vi "Pre Launch Init.vi"(11 "ATM-Controller in":refnum<class "ATM-Controller.lvclass">) -> (0 "error out":errorcluster, 3 "ATM-Controller out":refnum<class "ATM-Controller.lvclass">)   [LabVIEW 2025, in "ATM-Controller.lvlib" / "ATM-Controller.lvclass"]
doc: "<p>(<strong>Filename</strong>: <span class=\"dnl\">Actor Framework.lvlib:Actor.lvclass:Pre Launch Init.vi</span>)</p>\n<p>Defines behavior that occurs after the <a href=\"nihelplauncher://docs/csh?context=lvcore_lvcomm_af_launch_nested_actor\">Launch Nested Actor</a> method is invoked but before the actor's Actor Core method begins running.</p>\n<p>By default, this method does nothing. A descendant class may override it to define behavior.</p>"
uses:
  ATM-Controller.lvclass
  ATM-Controller.lvclass/ATM-Controller.ctl
  <vilib>/ActorFramework/Actor/Actor.lvclass
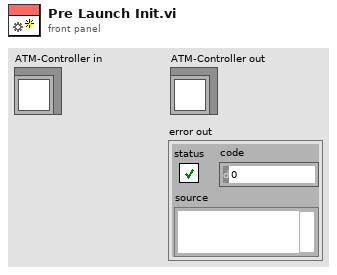
[diagram p1: front panel]
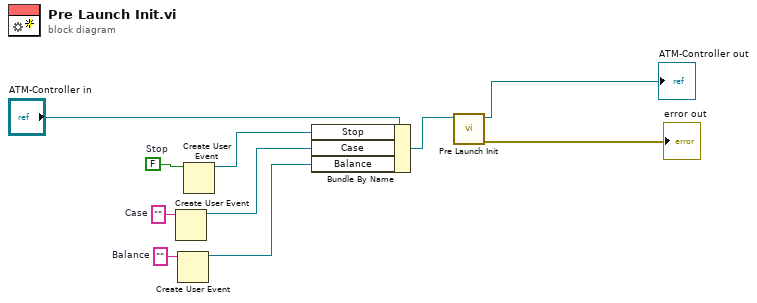
[diagram p0: block diagram]
diagram:
  w2 = ""  # Balance
  w4 = ""  # Case
  w7 = FALSE  # Stop
  n1 = Create User Event(user event datatype=w4) -> (user event=w3:refnum<user-event>)  [unwired: 1 in, 1 out]
  n2 = Create User Event(user event datatype=w2) -> (user event=w1:refnum<user-event>)  [unwired: 1 in, 1 out]
  n3 = Create User Event(user event datatype=w7) -> (user event=w5:refnum<user-event>)  [unwired: 1 in, 1 out]
  n4 = Bundle By Name(cluster="ATM-Controller in", "Stop"=w5, "Case"=w3, "Balance"=w1) -> (w6:refnum<class "ATM-Controller.lvclass">)
  n5 = call-parent "Pre Launch Init.vi"("Actor in"=w6) -> ("error out"=→"error out":errorcluster, "Actor out"=→"ATM-Controller out":refnum<class "ATM-Controller.lvclass">)  [unwired: 9 in]
